vi "Analogue 1 (Phase, Phase Shifter).vi"(11 "Phase Shifter":u32(knob) scale=0.0..3.0) -> (0 "Vps 6":fxp<+/-,23,10> format="%.2g", 1 "Vps 5":fxp<+/-,23,10> format="%.2g", 2 "Vps 4":fxp<+/-,23,10> format="%.2g", 3 "Vps 3":fxp<+/-,23,10> format="%.2g", 8 "Vps 2":fxp<+/-,23,10> format="%.2g", 9 "Vps 1":fxp<+/-,23,10> format="%.2g")   [LabVIEW 2023]
uses:
  <vilib>/rvi/eio/common/nirviEmuTemplateMethod_errors.vi
  <vilib>/eio/EIONode/EIONode.xnode
panel:
  # "Analogue 1: Phase Shifter, Phase"
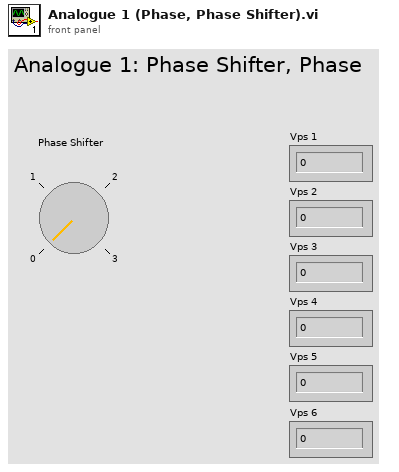
[diagram p1: front panel]
types:
  T1 = cluster{"ps 1":fxp<+/-,20,5>, "ps 2":fxp<+/-,20,5>, "ps 3":fxp<+/-,20,5>, "ps 4":fxp<+/-,20,5>, "ps 5":fxp<+/-,20,5>, "ps 6":fxp<+/-,20,5>}[]
  T2 = cluster{"ps 1":fxp<+/-,20,5>, "ps 2":fxp<+/-,20,5>, "ps 3":fxp<+/-,20,5>, "ps 4":fxp<+/-,20,5>, "ps 5":fxp<+/-,20,5>, "ps 6":fxp<+/-,20,5>}
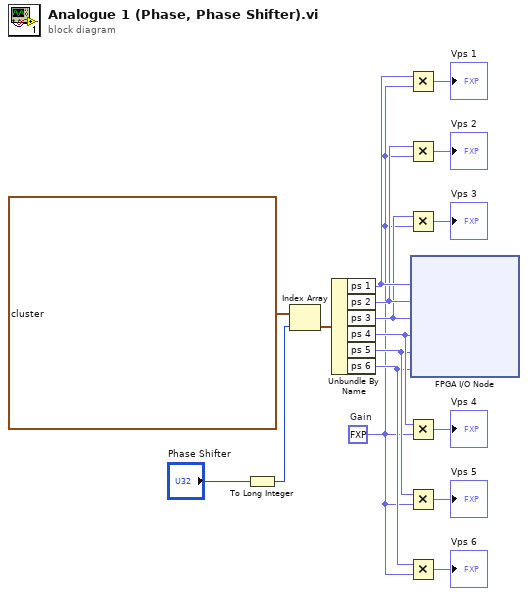
[diagram p0: block diagram]
diagram:
  w7 = fxp<+,3,5> 20.0  # Gain
  n1 = To Long Integer(number="Phase Shifter") -> (32bit integer=w15:i32)
  n2 = Index Array(array=T1 [{"ps 1"=0.0, "ps 2"=0.0, "ps 3"=0.0, "ps 4"=0.0, "ps 5"=0.0, "ps 6"=0.0}, {"ps 1"=0.0, "ps 2"=0.0, "ps 3"=0.0, "ps 4"=0.0, "ps 5"=0.0, "ps 6"=0.0}, {"ps 1"=0.0, "ps 2"=0.0, "ps 3"=0.0, "ps 4"=0.0, "ps 5"=0.0, "ps 6"=0.0}, {"ps 1"=0.0, "ps 2"=0.0, "ps 3"=0.0, "ps 4"=0.0, "ps 5"=0.0, "ps 6"=0.0}], index=w15) -> (element=w14:T2)
  n3 = Unbundle By Name(w14) -> ("ps 1"=w13:fxp<+/-,20,5>, "ps 2"=w12:fxp<+/-,20,5>, "ps 3"=w11:fxp<+/-,20,5>, "ps 4"=w10:fxp<+/-,20,5>, "ps 5"=w9:fxp<+/-,20,5>, "ps 6"=w8:fxp<+/-,20,5>)
  n4 = Multiply(x=w13, y=w7) -> (x*y=→"Vps 1":fxp<+/-,23,10>)
  n5 = Multiply(x=w12, y=w7) -> (x*y=→"Vps 2":fxp<+/-,23,10>)
  n6 = Multiply(x=w11, y=w7) -> (x*y=→"Vps 3":fxp<+/-,23,10>)
  n7 = Multiply(x=w10, y=w7) -> (x*y=→"Vps 4":fxp<+/-,23,10>)
  n8 = Multiply(x=w9, y=w7) -> (x*y=→"Vps 5":fxp<+/-,23,10>)
  n9 = Multiply(x=w8, y=w7) -> (x*y=→"Vps 6":fxp<+/-,23,10>)
  n10 = xnode "FPGA I/O Node"("Mod8/AO0"=w13, "Mod8/AO2"=w12, "Mod8/AO4"=w11, "Mod8/AO6"=w10, "Mod8/AO8"=w9, "Mod8/AO10"=w8) -> ()  [unwired: 6 in, 6 out]
